vi "GUI Waveform Show.vi"(8 "error in":errorcluster) -> (0 "error out":errorcluster)   [LabVIEW 2020]
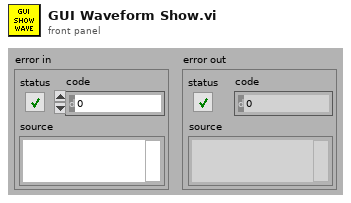
[diagram p1: front panel]
types:
  T1 = enum32{"Invalid", "Standard", "Closed", "Hidden", "Minimized", "Maximized"}
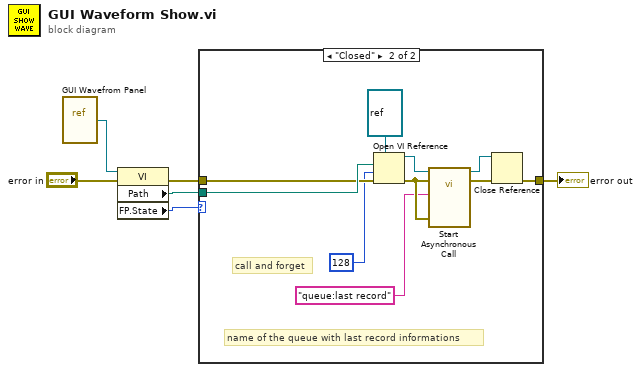
[diagram p0: block diagram]
diagram:
  n1 = vi-ref "GUI Wavefrom Panel.vi"() -> (w5:refnum<vi>)
  n2 = property class="VI"(reference=w5, error in="error in") -> (error out=w3:errorcluster, "Path"=w4:path, "FP.State"=w1:T1)  [unwired: 1 out]
  n3 = case shown="\"Closed\"" w1 {
    tunnel: w4 -> [_ w17]
    tunnel: w3 -> [w7 w16]
    tunnel: [w7 w9] -> w2
    frame Default {
    }
    frame "Closed" {
      # "name of the queue with last record informations"
      # "call and forget"
      n4 = Open VI Reference(type specifier VI Refnum (for type only)=refnum<vi> refnum, vi path=w17, options=128, error in (no error)=w16) -> (vi reference=w14:refnum<vi>, error out=w13:errorcluster)  [unwired: 2 in]
      n5 = call-by-ref "Start Asynchronous Call"(reference=w14, error in=w13, "error in"=w13, "source name ('last record')"="queue:last record") -> (reference out=w10:refnum<vi>, error out=w11:errorcluster)  [unwired: 9 in, 1 out]
      n6 = Close Reference(reference=w10, error in (no error)=w11) -> (error out=w9:errorcluster)
    }
  }
  "error out" <- w2
